vi "UI Initialize.vi"(8 "error in (no error)":errorcluster, 11 "GObject View in":refnum<class "Resource View.lvclass">) -> (0 "error out":errorcluster, 3 "GObject View out":refnum<class "Resource View.lvclass">)   [LabVIEW 2013, in "SET Project Editor.lvlib" / "Resource View.lvclass"]
uses:
  Resource View.lvclass
  MCListbox View/MCListbox View.lvclass
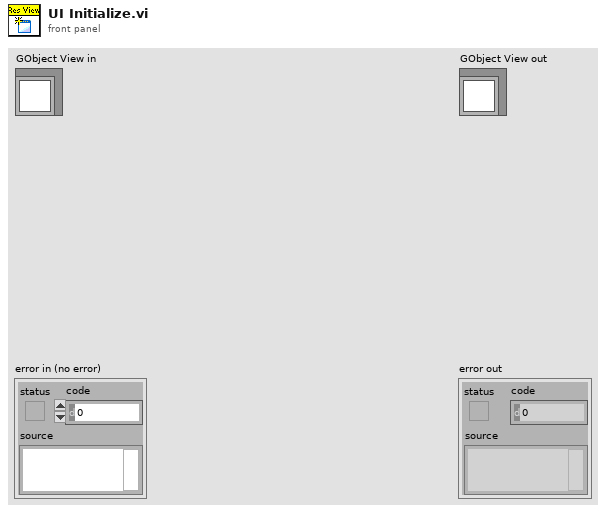
[diagram p1: front panel]
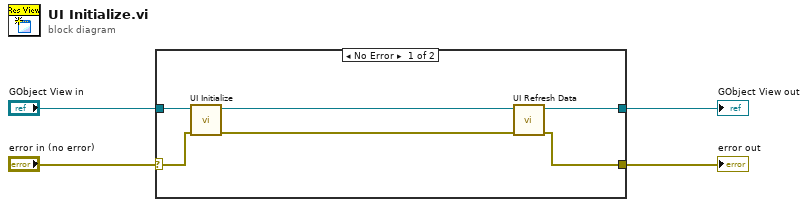
[diagram p0: block diagram]
diagram:
  n1 = case shown="No Error" "error in (no error)" {
    selector: "error in (no error)" -> [w9 w12]
    tunnel: [w5 w12] -> w3
    tunnel: [w6 w11] -> w1
    tunnel: "GObject View in" -> [w10 w11]
    frame No Error {
      n2 = call-parent "UI Initialize.vi"("error in (no error)"=w9, "View in"=w10) -> ("error out"=w7:errorcluster, "View out"=w8:refnum<class "Resource View.lvclass">)  [unwired: 8 in]
      n3 = call-dynamic "UI Refresh Data.vi"("error in (no error)"=w7, "Resource View in"=w8) -> ("error out"=w5:errorcluster, "Resource View out"=w6:refnum<class "Resource View.lvclass">)  [unwired: 8 in]
    }
    frame Error {
    }
  }
  "error out" <- w3
  "GObject View out" <- w1
